vi "exnFormulaBlock how many pts in the wave.vi"(0 "Array":waveform(dbl)[](array[waveform]), 1 "Boolean":bool, 2 "Iteration":i32) -> (3 "Waveform":waveform(dbl), 4 "Y":dbl[](array[numeric]) format="%0.2f", 5 "size(s)":i32, 6 "x = y?":bool)   [LabVIEW 2017]
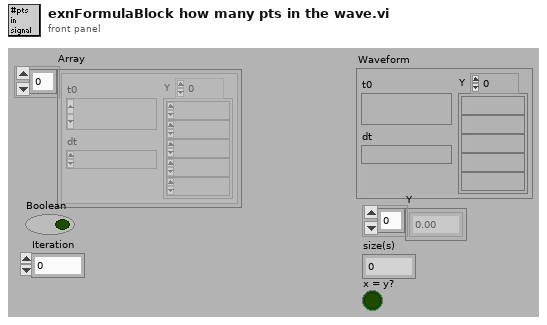
[diagram p1: front panel]
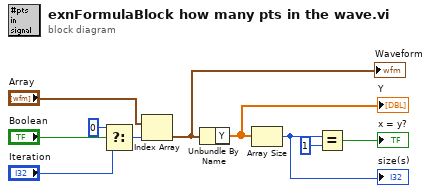
[diagram p0: block diagram]
diagram:
  n1 = Select(t=0, s="Boolean", f="Iteration") -> (s? t:f=w5:i32)
  n2 = Index Array(array="Array", index=w5) -> (element=w1:waveform(dbl))
  "Waveform" <- w1
  n3 = Unbundle By Name(w1) -> ("Y"=w10:dbl[])
  "Y" <- w10
  n4 = Array Size(array=w10) -> (size(s)=w6:i32)
  "size(s)" <- w6
  n5 = Equal?(x=w6, y=u8 1) -> (x = y?=→"x = y?":bool)
